vi "center calc.vi"(8 "Numeric 3":dbl) -> (3 "Numeric 4":dbl)   [LabVIEW 2016]
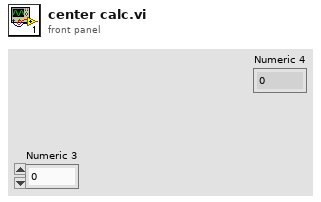
[diagram p1: front panel]
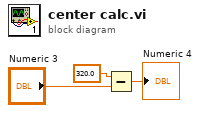
[diagram p0: block diagram]
diagram:
  n1 = Subtract(x=320.0, y="Numeric 3") -> (x-y=→"Numeric 4":dbl)
